vi "Send GCODE.vi"(8 "error in (no error)":errorcluster, 9 "String in":string, 10 "Message Data":variant, 11 "Cluster":T1) -> (0 "error out":errorcluster, 3 "String out":string)   [LabVIEW 2021]
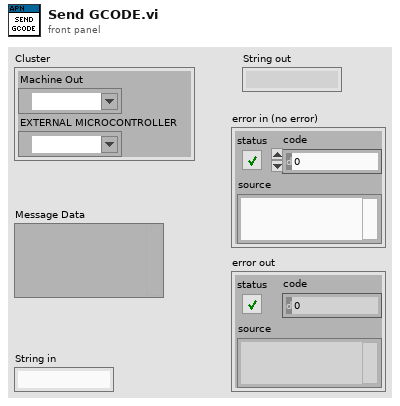
[diagram p1: front panel]
types:
  T1 = cluster{"Machine Out":refnum<visa-resource-name>, "EXTERNAL MICROCONTROLLER":refnum<visa-resource-name>}
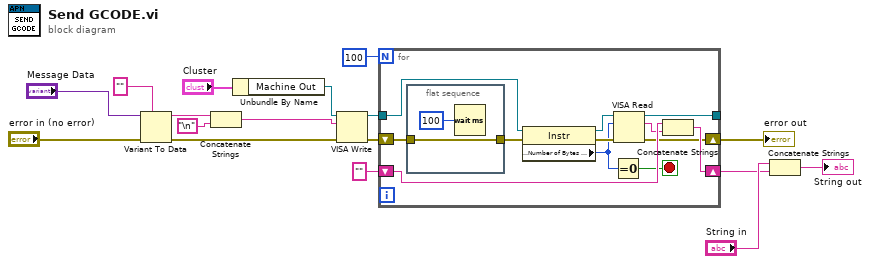
[diagram p0: block diagram]
diagram:
  n1 = Variant To Data(error in="error in (no error)", type="", Variant="Message Data") -> (data=w14:string, error out=w9:errorcluster)
  n2 = Concatenate Strings(w14, "\n") -> (w8:string)
  n3 = Unbundle By Name("Cluster") -> ("Machine Out"=w11:refnum<visa-resource-name>)
  n4 = VISA Write(VISA resource name=w11, write buffer=w8, error in (no error)=w9) -> (VISA resource name out=w4:refnum<visa-resource-name>, error out=w3:errorcluster)  [unwired: 1 out]
  n5 = for {
    N: 100 -> [_]
    tunnel: w4 -> [w26]
    shift-right: [w29] -> w15
    shift-left: "" -> [w28]
    shift-right: [w23] -> w13
    shift-left: w3 -> [w21]
    tunnel: [w18] -> _
    stop <- w19 stop-if-true
    n6 = flat-sequence {
      tunnel: w21 -> [w30]
      tunnel: [w30] -> w20
      frame #0 {
        n7 = Wait (ms)(milliseconds to wait=u32 100) -> ()  [unwired: 1 out]
      }
    }
    n8 = property class="Instr"(reference=w26, error in=w20) -> (reference out=w22:refnum<visa-resource-name>, error out=w27:errorcluster, "Serial Settings:Number of Bytes at Serial Port"=w24:u32)
    n9 = Equal To 0?(x=w24) -> (x = 0?=w19:bool)
    n10 = VISA Read(VISA resource name=w22, byte count=w24, error in (no error)=w27) -> (VISA resource name out=w18:refnum<visa-resource-name>, read buffer=w25:string, error out=w23:errorcluster)  [unwired: 1 out]
    n11 = Concatenate Strings(w28, w25) -> (w29:string)
  }
  "error out" <- w13
  n12 = Concatenate Strings("String in", w15) -> (→"String out":string)
